vi "executeDefensivePlay.vi"(8 "error in (no error)":errorcluster, 11 "Game in":refnum<class "Game.lvclass">) -> (0 "error out":errorcluster, 3 "Game out":refnum<class "Game.lvclass">)   [LabVIEW 2018, in "Game.lvclass"]
uses:
  Game.lvclass
  Game.lvclass/Game.ctl
  Team_class/Team.lvclass/Team.ctl
  Playbook_class/Playbook.lvclass/Playbook.ctl
  TestPlay_class/TestPlay.lvclass/TestPlay.ctl
  Robot_class/Robot.lvclass/Robot.ctl
  Robot_class/Read role.vi
  Playbook_class/Read defensive_plays.vi
  TestPlay_class/Read Roles.vi
  Read DefensiveTeam.vi
  Read Playbook.vi
  Team_class/Read RobotRef.vi
  Team_class/Read DefensivePlay.vi
  Team_class/Write RobotRef.vi
  Write DefensiveTeam.vi
  Ally_class/Ally.lvclass
  C:/Users/nicolas.oliveira/roboime/SSL_AI/Team_class/Team.lvclass
  Playbook_class/Playbook.lvclass
  Robot_class/Robot.lvclass
  Play_class/Play.lvclass
  TestPlay_class/TestPlay.lvclass
  TestRole_class/TestRole.lvclass
  Role_class/Role.lvclass
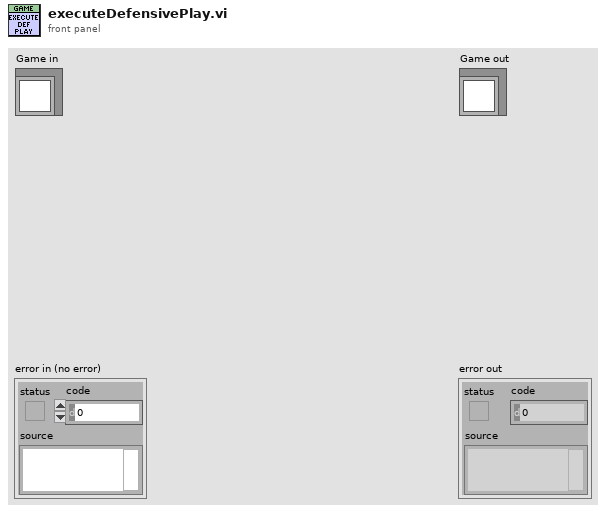
[diagram p1: front panel]
types:
  T1 = typedef "DefensivePlay.ctl" = enum16{"TestPlay", "Default", "Duelist", "Halt", "Timeout", "PenaltyEnemy", "PenaltyAlly"}
  T2 = cluster{"Play":refnum<class "Play.lvclass">, "TestPlay":refnum<class "TestPlay.lvclass">}
  T3 = typedef "roles.ctl" = enum16{"Halt", "Role", "TestRole"}
  T4 = cluster{"TestRole":refnum<class "TestRole.lvclass">, "Role":refnum<class "Role.lvclass">}
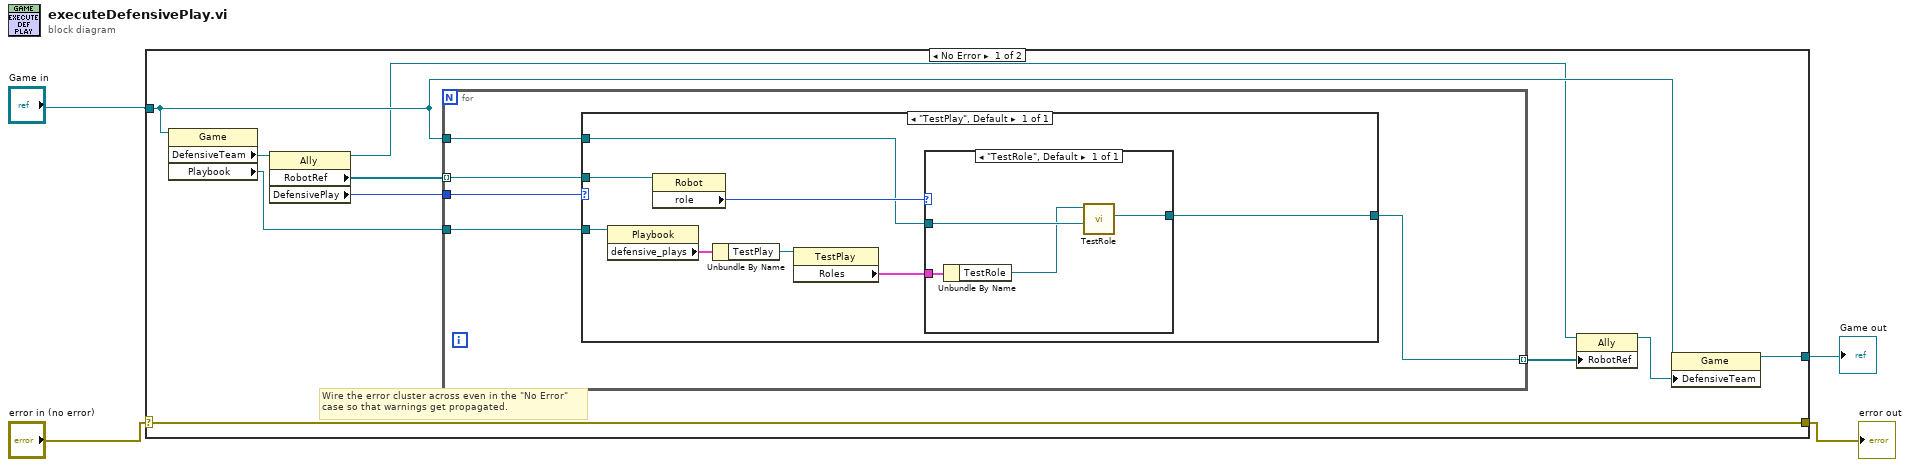
[diagram p0: block diagram]
diagram:
  n1 = case shown="No Error" "error in (no error)" {
    selector: "error in (no error)" -> [w14 w33]
    tunnel: [w14 w33] -> w1
    tunnel: [w6 w32] -> w2
    tunnel: "Game in" -> [w9 w32]
    frame No Error {
      # "Wire the error cluster across even in the \"No Error\"\ncase so that warnings get propagated."
      n2 = property class="Game"(reference=w9) -> ("DefensiveTeam"=w13:refnum<class "Ally.lvclass">, "Playbook"=w10:refnum<class "Playbook.lvclass">)  [unwired: 1 in, 2 out]
      n3 = property class="Ally"(reference=w13) -> (reference out=w8:refnum<class "Ally.lvclass">, "RobotRef"=w12:refnum<class "Robot.lvclass">[], "DefensivePlay"=w11:T1)  [unwired: 1 in, 1 out]
      n4 = for {
        tunnel: w12 -> [w17] mode=indexing
        tunnel: w11 -> [w19]
        tunnel: w10 -> [w18]
        tunnel: w9 -> [w16]
        tunnel: [w15] -> w7 mode=indexing
        n5 = case shown="\"TestPlay\", Default" w19 {
          tunnel: w18 -> [w27]
          tunnel: w17 -> [w24]
          tunnel: w16 -> [w21]
          tunnel: [w20] -> w15
          frame "TestPlay", Default {
            n6 = property class="Playbook"(reference=w27) -> ("defensive_plays"=w26:T2)  [unwired: 1 in, 2 out]
            n7 = property class="Robot"(reference=w24) -> ("role"=w23:T3)  [unwired: 1 in, 2 out]
            n8 = Unbundle By Name(w26) -> ("TestPlay"=w25:refnum<class "TestPlay.lvclass">)
            n9 = property class="TestPlay"(reference=w25) -> ("Roles"=w22:T4)  [unwired: 1 in, 2 out]
            n10 = case shown="\"TestRole\", Default" w23 {
              tunnel: w22 -> [w31]
              tunnel: w21 -> [w30]
              tunnel: [w29] -> w20
              frame "TestRole", Default {
                n11 = Unbundle By Name(w31) -> ("TestRole"=w28:refnum<class "TestRole.lvclass">)
                n12 = call-dynamic "TestRole.vi"("Game in"=w30, "TestRole in"=w28) -> ("Robot out"=w29:refnum<class "Robot.lvclass">)  [unwired: 6 in, 3 out]
              }
            }
          }
        }
      }
      n13 = property class="Ally"(reference=w8, "RobotRef"=w7) -> (reference out=w5:refnum<class "Ally.lvclass">)  [unwired: 1 in, 1 out]
      n14 = property class="Game"(reference=w9, "DefensiveTeam"=w5) -> (reference out=w6:refnum<class "Game.lvclass">)  [unwired: 1 in, 1 out]
    }
    frame Error {
    }
  }
  "error out" <- w1
  "Game out" <- w2
